vi "Example_Host_cRIO.vi"() -> ()   [LabVIEW 2011]
uses:
  <vilib>/rvi/interface/nirviOpenFPGA/nirviOpenFPGA.xnode
  Mezzanine DIO FPGA/SPI/spi_single port_example/FPGA Bitfiles/SPI Single Port Ex~B4_FPGA Target_FPGA_Top_Level_cRI~69.lvbit
  Mezzanine DIO FPGA/SPI/spi_single port_example/FPGA/FPGA_Top_Level_cRIO_Main.vi
  Host API/Controls/FPGA SPI_FPGA Ref.ctl
  <vilib>/rvi/interface/nirviCloseFPGA/nirviCloseFPGA.xnode
  Host API/Controls/FPGA SPI_SPI Configuration Cluster.ctl
panel:
  out "error out":errorcluster
  in  "stop":bool
  in  "Write Data":u8[](array[numeric])
  in  "Configuration Cluster":T1={"CS"=1, "Clock Rate (Hz)"=50000.0, "Clock Mode"=0, "CS Active State"=FALSE} {"CS" items=["0"=1, "1"=2, "2"=4, "3"=8, "4"=16, "5"=32, "6"=64, "7"=128]; "Clock Mode" items=["0", "1", "2", "3"]}
  in  "Total Bits":u16=8
  out "Read Data":u8[](array[numeric])
  in  "Write":bool
  # "Configure SPI"
  # "Write SPI"
  # "Control and Status"
  # "Read SPI"
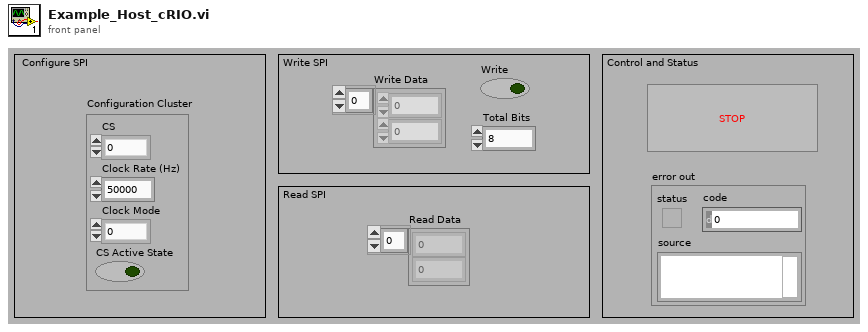
[diagram p1: front panel]
types:
  T1 = typedef "FPGA SPI_SPI Configuration Cluster.ctl" = cluster{"CS":u8, "Clock Rate (Hz)":dbl, "Clock Mode":u8, "CS Active State":bool}
  T2 = typedef "FPGA SPI_FPGA Ref.ctl" = refnum<k20>
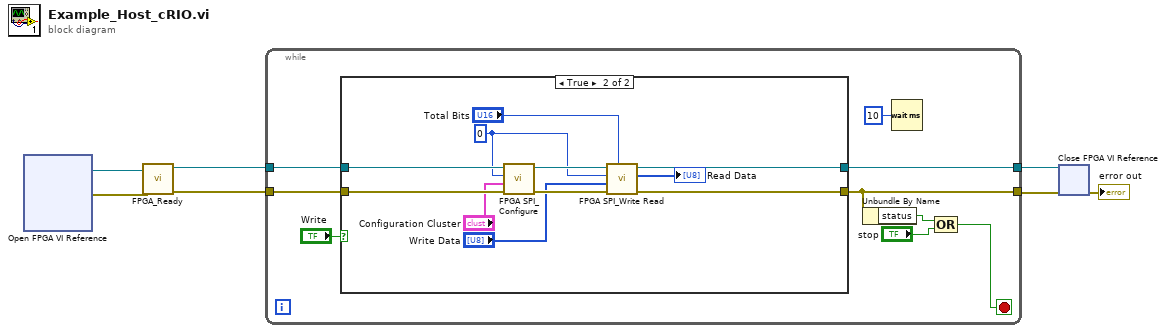
[diagram p0: block diagram]
diagram:
  n1 = xnode "Open FPGA VI Reference"() -> ("FPGA VI Reference Out"=w7:T2, "error out"=w6:errorcluster)  [unwired: 2 in]
  n2 = call "FPGA_Ready.vi"("Error In"=w6, "FPGA VI Reference In"=w7) -> ("Error Out"=w4:errorcluster, "FPGA VI Reference Out"=w5:T2)  [unwired: 7 out]
  n3 = while {
    tunnel: w5 -> [w16]
    tunnel: w4 -> [w15]
    tunnel: [w13] -> w3
    tunnel: [w12] -> w2
    stop <- w8 stop-if-true
    n4 = case shown="True" "Write" {
      tunnel: w16 -> [w18 w29]
      tunnel: w15 -> [w17 w27]
      tunnel: [w17 w25] -> w12
      tunnel: [w18 w24] -> w13
      frame False {
      }
      frame True {
        w20 = u8 0 ("Port")
        n5 = call "FPGA SPI_Configure.vi"("error in"=w27, "Configuration Cluster"="Configuration Cluster", "Port"=w20, "FPGA VI Reference"=w29) -> ("error out"=w26:errorcluster, "FPGA VI Reference Out"=w28:T2)  [unwired: 6 out]
        n6 = call "FPGA SPI_Write Read.vi"("Total Bits"="Total Bits", "error in"=w26, "Write Data"="Write Data", "Port"=w20, "FPGA VI Reference"=w28) -> ("error out"=w25:errorcluster, "Read Data"=→"Read Data":u8[], "FPGA VI Reference Out"=w24:T2)  [unwired: 4 out]
      }
    }
    n7 = Unbundle By Name(w12) -> ("status"=w10:bool)
    n8 = Wait (ms)(milliseconds to wait=u32 10) -> ()  [unwired: 1 out]
    n9 = Compound Arithmetic op=OR(w10, "stop") -> (w8:bool)
  }
  n10 = xnode "Close FPGA VI Reference"("FPGA VI Reference In"=w3, "error in"=w2) -> ("error out"=→"error out":errorcluster)
